vi "ULxTaskInfo.vi"(5 "task in":refnum<k24>, 6 "error in (no error)":errorcluster) -> (0 "task in 2":refnum<k24>, 1 "ToString":string, 2 "Task":i32, 3 "error out":errorcluster, 4 "NumberOfChannels":u32)   [LabVIEW 2010]
uses:
  C:/Program Files/National Instruments/LabVIEW 2010/vi.lib/ULx/ULx_LV.dll
  Program Files/National Instruments/LabVIEW 2010/vi.lib/ULx/ULx_LV.dll
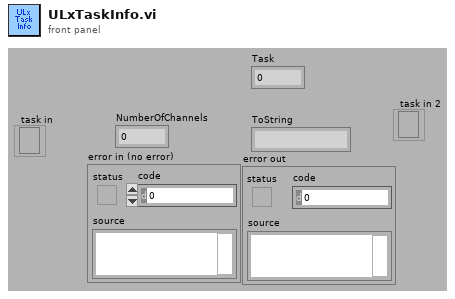
[diagram p1: front panel]
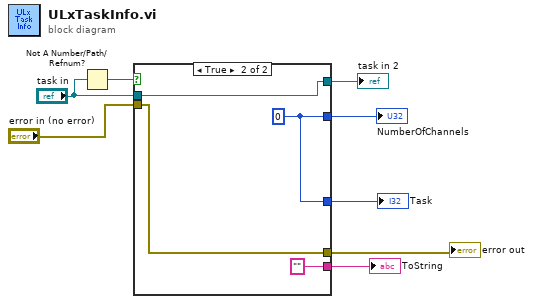
[diagram p0: block diagram]
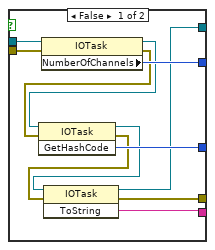
[diagram p2: hidden frame]
diagram:
  n1 = Not A Number/Path/Refnum?(number/path/refnum="task in") -> (NaN/Path/Refnum?=w7:bool)
  n2 = case shown="True" w7 {
    tunnel: "task in" -> [w19 w20]
    tunnel: [w18 w23] -> w8
    tunnel: [w16 w23] -> w5
    tunnel: [w14 "" ("ToString")] -> w4
    tunnel: [w13 w21] -> w3
    tunnel: "error in (no error)" -> [w12 w21]
    tunnel: [w11 w20] -> w2
    frame False {
      n3 = property class="IOTask"(reference=w19, error in=w12) -> (reference out=w17:refnum<k24>, error out=w9:errorcluster, "NumberOfChannels"=w18:u32)
      n4 = invoke class="IOTask" method="GetHashCode"(reference=w17, error in=w9) -> (reference out=w15:refnum<k24>, error out=w10:errorcluster, "GetHashCode"=w16:i32)  [unwired: 1 in]
      n5 = invoke class="IOTask" method="ToString"(reference=w15, error in=w10) -> (reference out=w11:refnum<k24>, error out=w13:errorcluster, "ToString"=w14:string)  [unwired: 1 in]
    }
    frame True {
      w23 = 0 ("NumberOfChannels")
    }
  }
  "NumberOfChannels" <- w8
  "Task" <- w5
  "ToString" <- w4
  "error out" <- w3
  "task in 2" <- w2
